vi "xcamera-make_balance-white-auto.vi"(11 "Option":enum16{"Off", "Once", "Continuous", "Stop"}(ring)) -> (3 "Serial String":string)   [LabVIEW 2012]
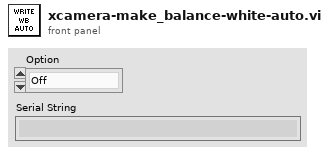
[diagram p1: front panel]
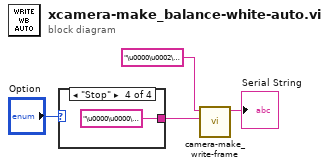
[diagram p0: block diagram]
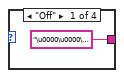
[diagram p2: hidden frame]
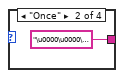
[diagram p3: hidden frame]
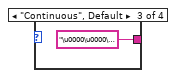
[diagram p4: hidden frame]
diagram:
  n1 = case shown="\"Stop\"" "Option" {
    tunnel: ["\u0000\u0000\u0000\u0001" ("Address") "\u0000\u0000\u0000\u0001" ("Address") "\u0000\u0000\u0000\u0002" ("Address") "\u0000\u0000\u0000\u0003" ("Address")] -> w1
    frame "Off" {
    }
    frame "Once" {
    }
    frame "Continuous", Default {
    }
    frame "Stop" {
    }
  }
  n2 = call "camera-make_write-frame.vi"("Data"=w1, "Address"="\u0000\u0002\u0004\u0000") -> ("Serial String"=→"Serial String":string)  [unwired: 9 in]
